vi "Teleop_Set_DrivingMode.vi"(11 "DrivingMode":i32) -> ()   [LabVIEW 2019]
uses:
  Teleop_Globals.vi
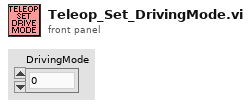
[diagram p1: front panel]
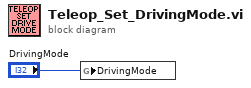
[diagram p0: block diagram]
diagram:
  n1 = global write "Teleop_Globals.vi" "DrivingMode"("DrivingMode") -> ()
